vi "Stitching-Resize stitched image.vi"(7 "Stitched image setup":T1, 8 "error in (no error)":errorcluster, 11 "Stitched image ref in":T2) -> (0 "error out":errorcluster, 3 "Stitched image ref":T2)   [LabVIEW 2020]
uses:
  <vilib>/vision/Image Controls.llb/IMAQ Image.ctl
  <vilib>/vision/NI_Vision_Development_Module.lvlib
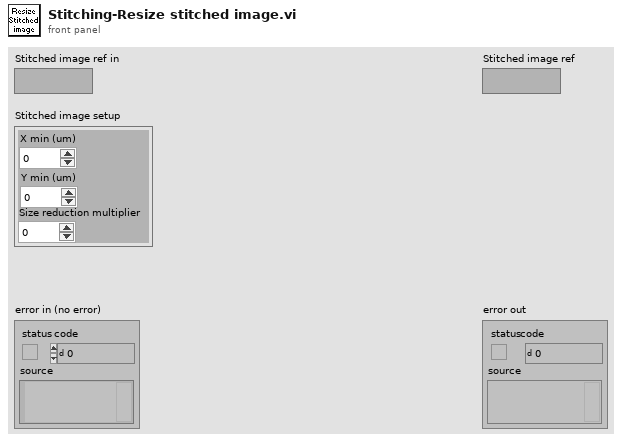
[diagram p1: front panel]
types:
  T1 = cluster{"X min (um) ":i32, "Y min (um)":i32, "Size reduction multiplier":dbl}
  T2 = typedef "IMAQ Image.ctl" = refnum<image>
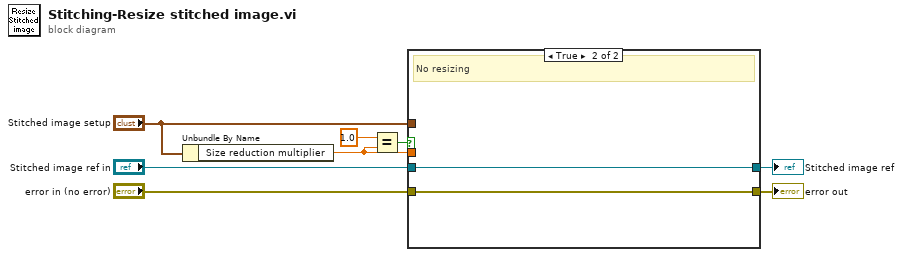
[diagram p0: block diagram]
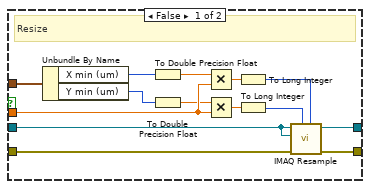
[diagram p2: hidden frame]
diagram:
  n1 = Unbundle By Name("Stitched image setup") -> ("Size reduction multiplier"=w1:dbl)
  n2 = Equal?(x=1.0, y=w1) -> (x = y?=w3:bool)
  n3 = case shown="True" w3 {
    tunnel: "Stitched image setup" -> [w22 _]
    tunnel: w1 -> [w19 _]
    tunnel: "Stitched image ref in" -> [w14 w24]
    tunnel: [w11 w24] -> w7
    tunnel: "error in (no error)" -> [w10 w23]
    tunnel: [w9 w23] -> w5
    frame False {
      # "Resize"
      n4 = Unbundle By Name(w22) -> ("X min (um)"=w21:i32, "Y min (um)"=w20:i32)
      n5 = To Double Precision Float(number=w21) -> (double precision float=w16:dbl)
      n6 = To Double Precision Float(number=w20) -> (double precision float=w15:dbl)
      n7 = Multiply(x=w16, y=w19) -> (x*y=w18:dbl)
      n8 = Multiply(x=w15, y=w19) -> (x*y=w17:dbl)
      n9 = To Long Integer(number=w18) -> (32bit integer=w13:i32)
      n10 = To Long Integer(number=w17) -> (32bit integer=w12:i32)
      n11 = call "IMAQ Resample"("X Resolution"=w13, "Y Resolution"=w12, "error in (no error)"=w10, "Image Dst"=w14, "Image Src"=w14) -> ("error out"=w9:errorcluster, "Image Dst Out"=w11:T2)  [unwired: 5 in]
    }
    frame True {
      # "No resizing"
    }
  }
  "Stitched image ref" <- w7
  "error out" <- w5
